vi "Pre Launch Init.vi"(11 "Main Display in":refnum<class "Main Display.lvclass">) -> (0 "error out":errorcluster, 3 "Main Display out":refnum<class "Main Display.lvclass">)   [LabVIEW 2016, in "Assert API Components.lvlib" / "Assert Display.lvlib" / "Main Display.lvlib" / "Main Display.lvclass"]
doc: "(<B>Filename</B>: Actor Framework.lvlib:Actor.lvclass:Pre Launch Init.vi)\n\nDefines behavior that occurs after the Launch Nested Actor method is invoked but before the actor's Actor Core method begins running.\n\nBy default, this method does nothing. A descendant class may override it to define behavior."
uses:
  Main Display.lvclass
  Display Configurations/Standard Display Configuration/Standard Display Configuration.lvclass
  D:/Work/Projects/Actor_Assert_API/Main Display/Display Configurations/Base Display Configuration.lvclass
  Main Display.lvclass/Main Display.ctl
  Base UI Component/Base UI Component/Base UI Component.lvclass
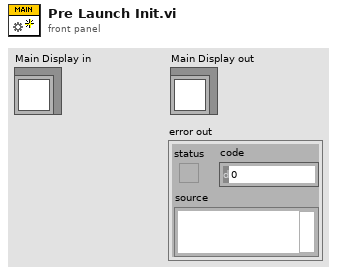
[diagram p1: front panel]
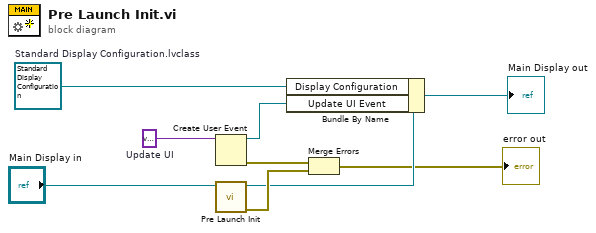
[diagram p0: block diagram]
diagram:
  w1 = refnum<class "Standard Display Configuration.lvclass"> refnum  # Standard Display Configuration.lvclass
  w6 = variant  # Update UI
  n1 = Create User Event(user event datatype=w6) -> (user event=w4:refnum<user-event>, error out=w2:errorcluster)  [unwired: 1 in]
  n2 = call-parent "Pre Launch Init.vi"("Base UI Component in"="Main Display in") -> ("error out"=w9:errorcluster, "Base UI Component out"=w8:refnum<class "Main Display.lvclass">)  [unwired: 9 in]
  n3 = Bundle By Name(cluster=w8, "Display Configuration"=w1, "Update UI Event"=w4) -> (→"Main Display out":refnum<class "Main Display.lvclass">)
  n4 = Merge Errors(w2, w9) -> (→"error out":errorcluster)
